vi "Pre Launch Init.vi"(11 "Ex Nested in":refnum<class "SuperActor.lvclass">) -> (0 "error out":errorcluster, 3 "Ex Nested out":refnum<class "SuperActor.lvclass">)   [LabVIEW 2014, in "SuperActor.lvclass"]
doc: "(<B>Filename</B>: Actor Framework.lvlib:Actor.lvclass:Pre Launch Init.vi)\n\nDefines behavior that occurs after the Launch Nested Actor method is invoked but before the actor's Actor Core method begins running.\n\nBy default, this method does nothing. A descendant class may override it to define behavior."
uses:
  SuperActor.lvclass
  reusable/Session APIs/File Access/Config Data/Config Data.lvclass
  reusable/Session APIs/Session Log/System Log.lvclass
  reusable/Session APIs/File Access/Config Data/Config Data.lvclass/Config Data.ctl
  reusable/Session APIs/Session Log/System Log.lvclass/System Log.ctl
  SuperActor.lvclass/SuperActor.ctl
  reusable/Session APIs/File Access/Config Data/Accessors/Write Cfg Path.vi
  reusable/Session APIs/Session Log/Accessors/Write Main Path.vi
  reusable/Session APIs/Session Log/Accessors/Write Log Warnings_.vi
  reusable/Session APIs/Session Log/Accessors/Write Codes.vi
  reusable/Session APIs/File Access/Config Data/Accessors/Read Ref.vi
  Controller/xGlobal Data.vi
  <vilib>/Utility/config.llb/Read Key (Path).vi
  <vilib>/Utility/config.llb/Read Key (String).vi
  <vilib>/Utility/config.llb/Read Key (Boolean).vi
  <userlib>/_Session Fwk/Session - Root.lvclass
  <vilib>/Utility/config.llb/NI_LVConfig.lvlib
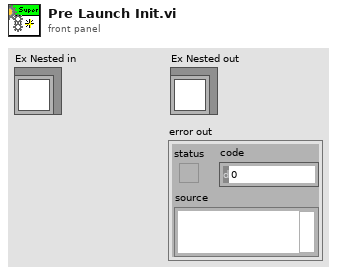
[diagram p1: front panel]
types:
  T1 = typedef "Session - Root.lvclass/Session Handle.ctl" = refnum<data-value>
  T2 = typedef "NI_LVConfig.lvlib/Config Data RefNum.ctl" = refnum<k1>
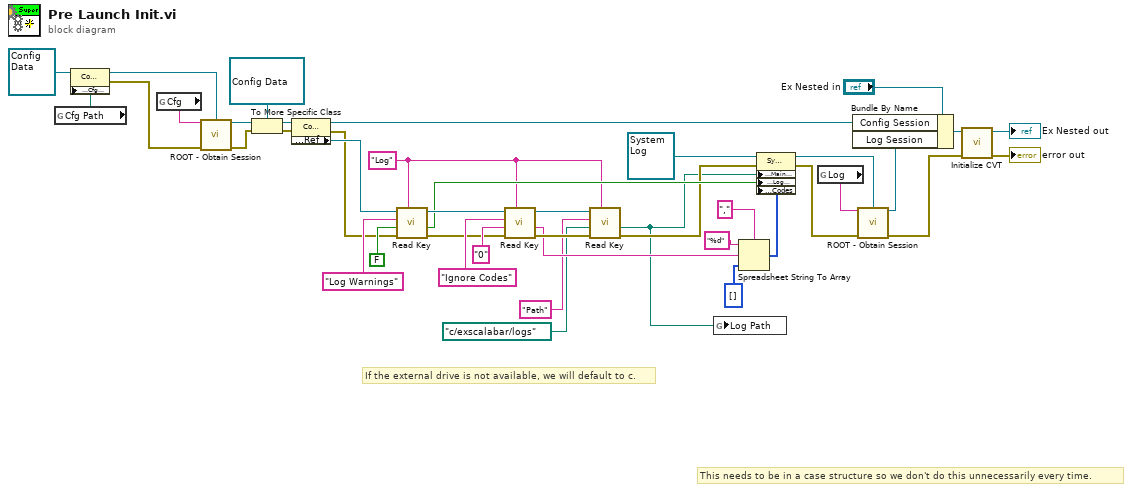
[diagram p0: block diagram]
diagram:
  w5 = "Log" ("section")
  # "If the external drive is not available, we will default to c."
  # "This needs to be in a case structure so we don't do this unnecessarily every time."
  n1 = global read "xGlobal Data.vi" "Cfg Path"() -> (w40:path)
  n2 = property class="Config Data"(reference=refnum<class "Config Data.lvclass"> refnum ("Config Data"), "Accessors:Cfg Path"=w40) -> (reference out=w21:refnum<class "Config Data.lvclass">, error out=w36:errorcluster)  [unwired: 1 in]
  n3 = global read "xGlobal Data.vi" "Cfg"() -> (w42:string)
  n4 = call <userlib>:"ROOT - Obtain Session.vi"("Session Name ()"=w42, "OBJ - Session"=w21, "error in (no error)"=w36) -> ("Session Handle"=w16:T1, "error out"=w9:errorcluster)  [unwired: 10 in, 1 out]
  n5 = To More Specific Class(target class=refnum<data-value> refnum, reference=w16, error in=w9) -> (specific class reference=w14:refnum<data-value>, error out=w13:errorcluster)
  n6 = property class="Config Data"(reference=w14, error in=w13) -> (reference out=w11:refnum<data-value>, error out=w10:errorcluster, "Accessors:Ref"=w12:T2)
  n7 = call-poly <vilib>:"Read Key.vi"("section"=w5, "error in (no error)"=w10, "default value"=FALSE, "key"="Log Warnings", "refnum"=w12) -> ("error out"=w26:errorcluster, "value"=w24:bool, "refnum out"=w25:T2)  [unwired: 3 in, 1 out]
  n8 = call-poly <vilib>:"Read Key.vi"("section"=w5, "error in (no error)"=w26, "default value"="0", "key"="Ignore Codes", "refnum"=w25) -> ("error out"=w8:errorcluster, "value"=w7:string, "refnum out"=w6:T2)  [unwired: 3 in, 1 out]
  n9 = call-poly <vilib>:"Read Key.vi"("section"=w5, "error in (no error)"=w8, "default value"=path "c:/exscalabar/logs" ("Log Path"), "key"="Path", "refnum"=w6) -> ("error out"=w3:errorcluster, "value"=w2:path)  [unwired: 3 in, 2 out]
  n10 = global write "xGlobal Data.vi" "Log Path"(w2) -> ()
  n11 = Spreadsheet String To Array(delimiter (Tab)=",", format string="%d", spreadsheet string=w7, array type (2D Dbl)=i32[] []) -> (array=w32:i32[])
  n12 = property class="Sys Log"(reference=refnum<class "System Log.lvclass"> refnum ("Sys Log"), error in=w3, "Accessors:Main Path"=w2, "Accessors:Log Warnings_"=w24, "Accessors:Codes"=w32) -> (reference out=w38:refnum<class "System Log.lvclass">, error out=w37:errorcluster)
  n13 = global read "xGlobal Data.vi" "Log"() -> (w39:string)
  n14 = call <userlib>:"ROOT - Obtain Session.vi"("Session Name ()"=w39, "OBJ - Session"=w38, "error in (no error)"=w37) -> ("Session Handle"=w33:T1, "error out"=w18:errorcluster)  [unwired: 10 in, 1 out]
  n15 = Bundle By Name(cluster="Ex Nested in", "Config Session"=w11, "Log Session"=w33) -> (w20:refnum<class "SuperActor.lvclass">)
  n16 = call-dynamic "Initialize CVT.vi"("error in"=w18, "Ex Nested in"=w20) -> ("error out"=→"error out":errorcluster, "Ex Nested out"=→"Ex Nested out":refnum<class "SuperActor.lvclass">)  [unwired: 8 in]
